vi "Execute Command.vi"(0 "SLSC Local in":refnum<class "SLSC Local.lvclass">, 5 "resources":string, 7 "command":refnum<k21>, 11 "error in (no error)":errorcluster, 12 "timeout (10 sec)":dbl=10.0) -> (4 "SLSC Local out":refnum<class "SLSC Local.lvclass">, 15 "error out":errorcluster)   [LabVIEW 2015, in "SLSC Local.lvclass"]
uses:
  SLSC Local.lvclass
  <vilib>/SLSC/SLSC.lvlib
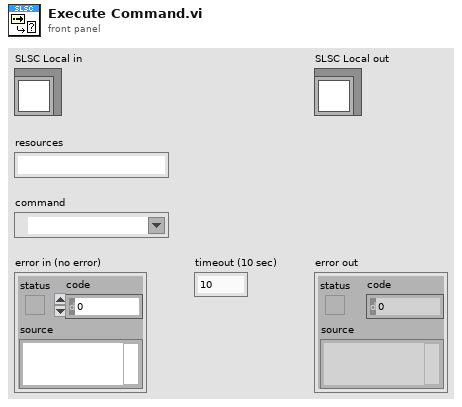
[diagram p1: front panel]
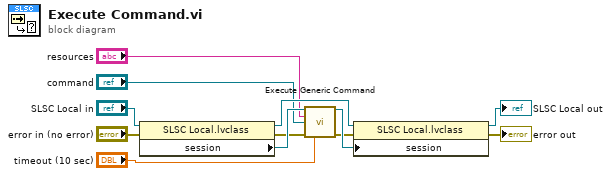
[diagram p0: block diagram]
diagram:
  n1 = property class="SLSC Local.lvclass"(reference="SLSC Local in", error in="error in (no error)") -> (reference out=w11:refnum<class "SLSC Local.lvclass">, error out=w4:errorcluster, "session"=w9:refnum<k21>)
  n2 = call <vilib>:"Execute Generic Command.vi"("session in"=w9, "resources"="resources", "command"="command", "error in (no error)"=w4, "timeout (10 sec)"="timeout (10 sec)") -> ("session out"=w8:refnum<k21>, "error out"=w3:errorcluster)  [unwired: 9 in]
  n3 = property class="SLSC Local.lvclass"(reference=w11, error in=w3, "session"=w8) -> (reference out=→"SLSC Local out":refnum<class "SLSC Local.lvclass">, error out=→"error out":errorcluster)
